vi "Multiplier_for_Voltage_Drift.vi"(9 "Voltage Read":dbl format="%_6g", 11 "Voltage Set":dbl format="%.6g") -> (2 "Multiplier":dbl)   [LabVIEW 2020]
panel:
  out "32bit integer":i32
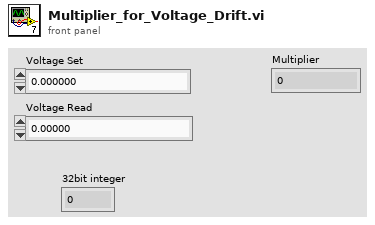
[diagram p1: front panel]
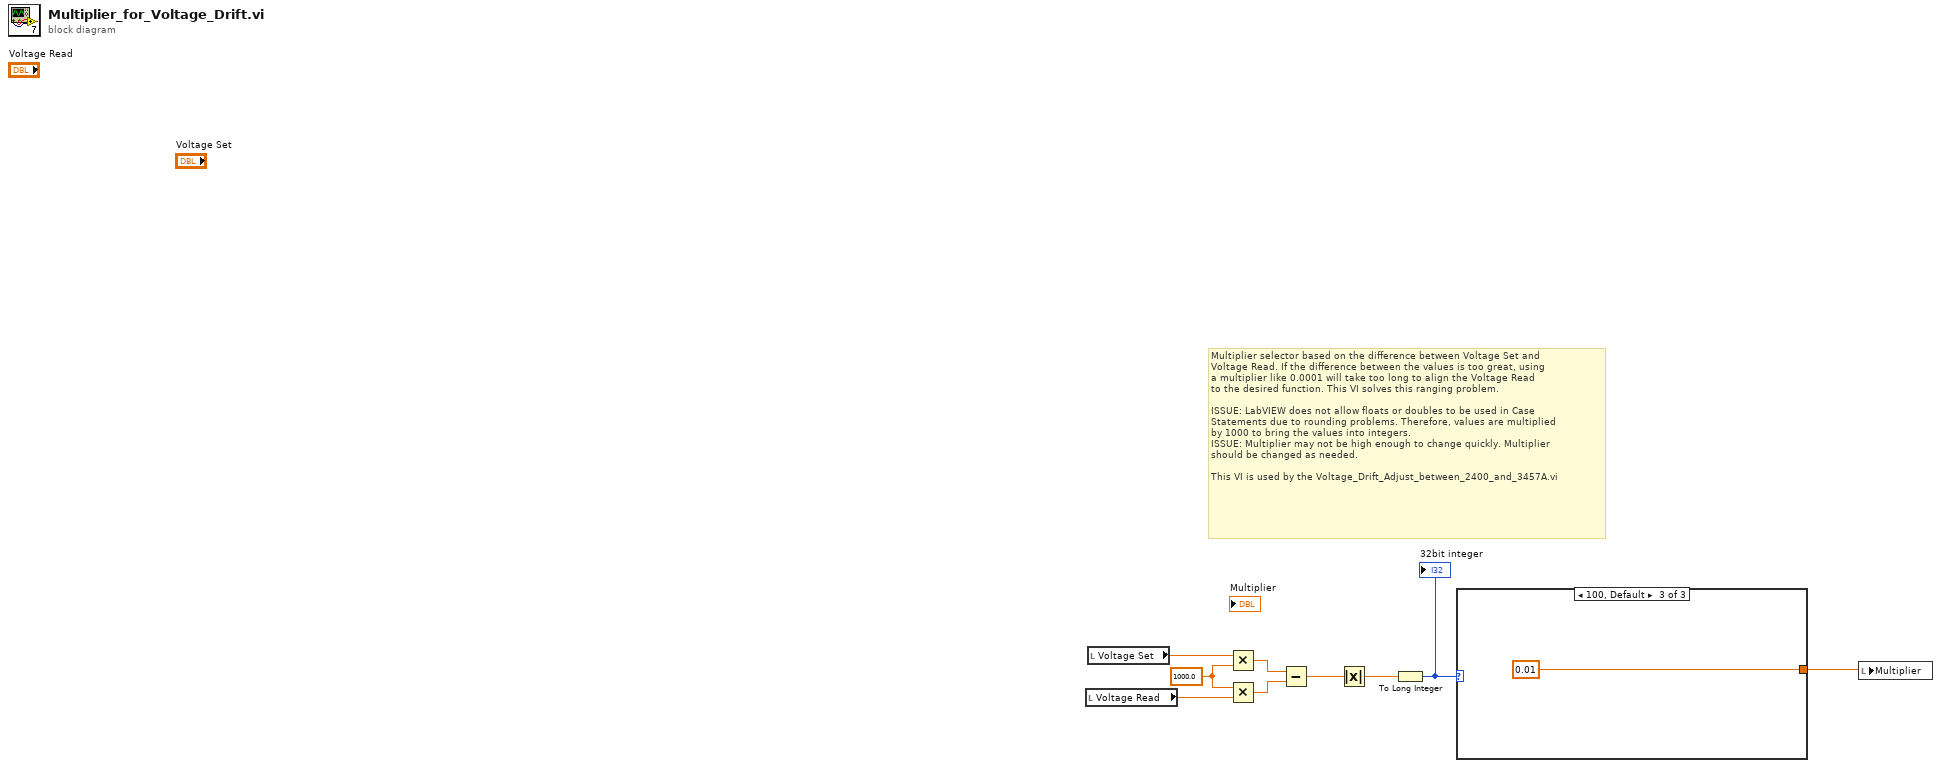
[diagram p0: block diagram]
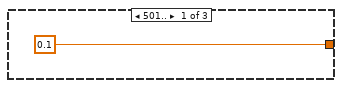
[diagram p2: hidden frame]
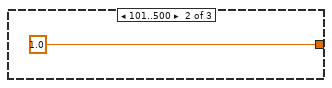
[diagram p3: hidden frame]
diagram:
  w7 = 1000.0 ("y")
  # "Multiplier selector based on the difference between Voltage Set and\nVoltage Read. If the difference between the values is too great, using\na multiplier like 0.0001 will take too long to align the Voltage Read\nto the desired function. This VI solves this ranging problem.\n\nISSUE: LabVIEW does not allow floats or doubles to be used in Case\nStatements due to rounding problems. Therefore, values are multiplied\nby 1000 to bring the values into integers.\nISSUE: Multiplier may not be high enough to change quickly. Multiplier\nshould be changed as needed.\n\nThis VI is used by the Voltage_Drift_Adjust_between_2400_and_3457A.vi"
  n1 = local read "Voltage Read"() -> (w8:dbl)
  n2 = local read "Voltage Set"() -> (w9:dbl)
  n3 = Multiply(x=w9, y=w7) -> (x*y=w6:dbl)
  n4 = Multiply(x=w7, y=w8) -> (x*y=w5:dbl)
  n5 = Subtract(x=w6, y=w5) -> (x-y=w2:dbl)
  n6 = Absolute Value(x=w2) -> (abs(x)=w1:dbl)
  n7 = To Long Integer(number=w1) -> (32bit integer=w4:i32)
  "32bit integer" <- w4
  n8 = case shown="100, Default" w4 {
    tunnel: [0.1 ("Multiplier") 1.0 ("Multiplier") 0.01 ("Multiplier")] -> w3
    frame 501.. {
    }
    frame 101..500 {
    }
    frame 100, Default {
    }
  }
  n9 = local write "Multiplier"(w3) -> ()
